vi "6.1. 通过匹配模式提取数字.vi"(10 "字符串":string="yi 2 -3 4.0 5.5") -> (2 "提取的数字":dbl[](array[numeric]) format="%#.6g")   [LabVIEW 2018]
doc: "通过“匹配模式”函数查找给定字符串中的所有数字，并以数组的方式返回。可识别的格式包括：\n\n123 1.23 .123 0.123 -1.23\n\n数字内不可出现空格或其他字符，但数字前后可出现任意字符。本范例假定输入字符串的小数分隔号为句号，而不是逗号。"
panel:
  # "概述：演示使用匹配模式函数从字符串提取数值的方法。\n操作步骤：\n1.指定一个包含数字的字符串的值。\n2.运行VI。“字符串”中的所有数字将显示在提取的数字数组中。"
  # "注：本范例不支持拼写出的数字（如上字符串中的\"yi\"）。同时也不支持科学计数法。此外，本范例仅从使用句点(.)作为小数点分隔符的字符串中提取十进制数。"
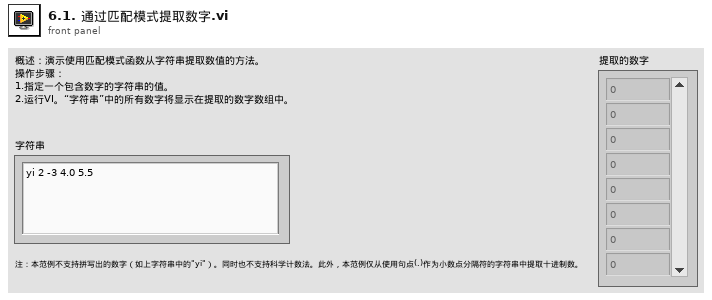
[diagram p1: front panel]
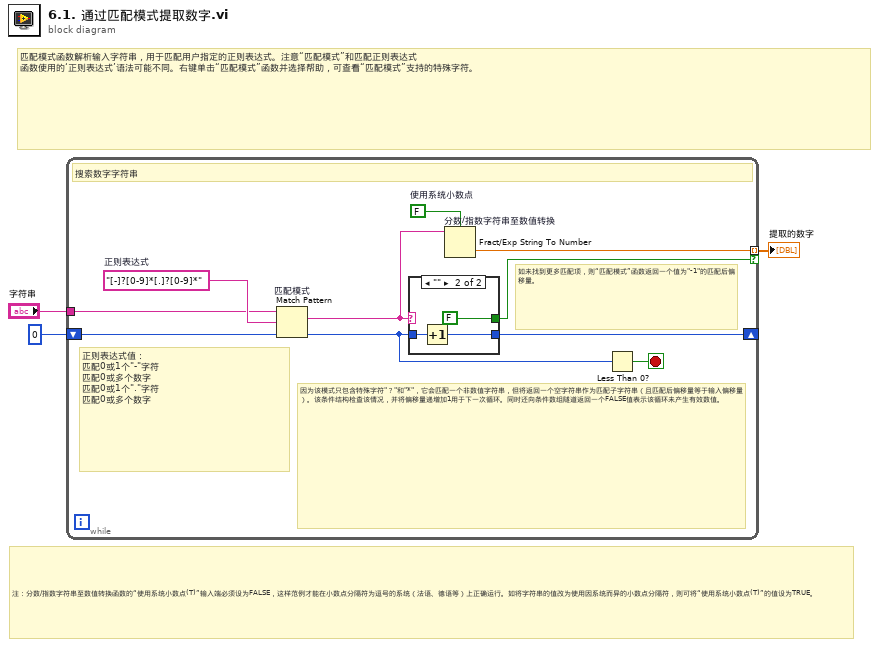
[diagram p0: block diagram]
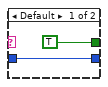
[diagram p2: hidden frame]
diagram:
  # "注：分数/指数字符串至数值转换函数的“使用系统小数点(T)”输入端必须设为FALSE，这样范例才能在小数点分隔符为逗号的系统（法语、德语等）上正确运行。如将字符串的值改为使用因系统而异的小数点分隔符，则可将“使用系统小数点(T)”的值设为TRUE。"
  # "匹配模式函数解析输入字符串，用于匹配用户指定的正则表达式。注意“匹配模式”和匹配正则表达式 函数使用的‘正则表达式’语法可能不同。右键单击“匹配模式”函数并选择帮助，可查看“匹配模式”支持的特殊字符。"
  n1 = while {
    shift-left: 0 -> [w9]
    shift-right: [w4] -> _
    tunnel: [w13] -> w3 mode=indexing if=w6
    tunnel: "字符串" -> [w8]
    stop <- w12 stop-if-true
    w11 = FALSE  # 使用系统小数点
    w10 = "[-]?[0-9]*[.]?[0-9]*"  # 正则表达式
    # "如未找到更多匹配项，则“匹配模式”函数返回一个值为\"-1\"的匹配后偏移量。"
    # "因为该模式只包含特殊字符\"？\"和\"*\"，它会匹配一个非数值字符串，但将返回一个空字符串作为匹配子字符串（且匹配后偏移量等于输入偏移量）。该条件结构检查该情况，并将偏移量递增加1用于下一次循环。同时还向条件数组隧道返回一个FALSE值表示该循环未产生有效数值。"
    # "正则表达式值：\n匹配0或1个\"-\"字符\n匹配0或多个数字\n匹配0或1个\".\"字符\n匹配0或多个数字"
    # "搜索数字字符串"
    n2 = Match Pattern "匹配模式"(string=w8, regular expression=w10, offset (0)=w9) -> (match substring=w7:string, offset past match=w5:i32)  [unwired: 2 out]
    n3 = case shown="\"\"" w7 {
      tunnel: [w15 w17] -> w4
      tunnel: [TRUE FALSE] -> w6
      tunnel: w5 -> [w15 w18]
      frame Default {
      }
      frame "" {
        n4 = Increment(x=w18) -> (x+1=w17:i32)
      }
    }
    n5 = Fract/Exp String To Number "分数/指数字符串至数值转换"(use system decimal point (T)=w11, string=w7) -> (number=w13:dbl)  [unwired: 2 in, 1 out]
    n6 = Less Than 0?(x=w5) -> (x < 0?=w12:bool)
  }
  "提取的数字" <- w3
